vi "GE 5565PIORC.Registers.DMASIZ0.DMA Transfer Size.Set.vi"(8 "error in (no error)":errorcluster, 10 "DMA Transfer Size (Bytes)":u32, 11 "GE 5565PIORC in":refnum<class "GE 5565PIORC.lvclass">) -> (0 "error out":errorcluster, 3 "GE 5565PIORC out":refnum<class "GE 5565PIORC.lvclass">)   [LabVIEW 2017, in "GE 5565PIORC.lvclass"]
doc: "Indicates the number of bytes to transfer during a DMA operation."
uses:
  GE 5565PIORC.lvclass
  GE 5565PIORC.Registers.Local Configuration.ctl
  GE 5565PIORC.lvclass/GE 5565PIORC.ctl
  GE 5565PIORC.Registers.Local Configuration.Read (U32).vi
  GE 5565PIORC.Registers.Local Configuration.Write (U32).vi
  Methods/GE 5565PIORC.Registers.Read.vi
  Methods/GE 5565PIORC.Registers.Read (U32).vi
  Methods/GE 5565PIORC.Registers.Write.vi
  Methods/GE 5565PIORC.Registers.Write (U32).vi
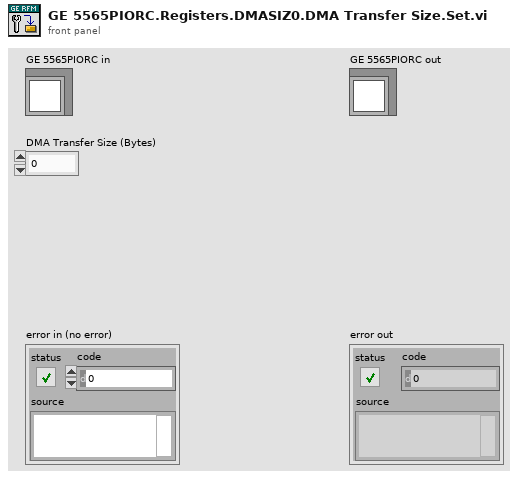
[diagram p1: front panel]
types:
  T1 = typedef "GE 5565PIORC.lvclass/GE 5565PIORC.Registers.Local Configuration.ctl" = u32
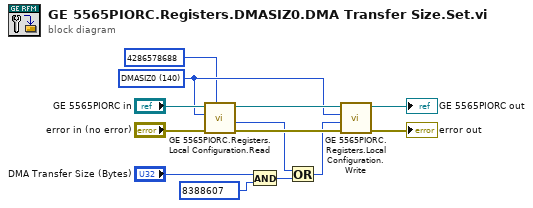
[diagram p0: block diagram]
diagram:
  w7 = T1 140 items=["MARBR"=8, "BIGEND"=12, "INTCSR"=104, "PCIHREV"=116, "DMAMODE0"=128, "DMAPADR0"=132, "DMALADR0"=136, "DMASIZ0"=140, "DMADPR0"=144, "DMACSR0"=168, "DMADAC0"=180, "LAS1RR"=240, "LAS1BA"=244] ("Local Configuration Registers")
  n1 = call-poly "GE 5565PIORC.Registers.Local Configuration.Read.vi"("Mask (0xFFFFFFFF)"=u32 4286578688, "error in (no error)"="error in (no error)", "Register"=w7, "GE 5565PIORC in"="GE 5565PIORC in") -> ("error out"=w13:errorcluster, "Value"=w3:u32, "GE 5565PIORC out"=w10:refnum<class "GE 5565PIORC.lvclass">)  [unwired: 5 in]
  n2 = And(x="DMA Transfer Size (Bytes)", y=u32 8388607 ("Mask (0xFFFFFFFF)")) -> (x .and. y?=w1:u32)
  n3 = Or(x=w3, y=w1) -> (x .or. y?=w2:u32)
  n4 = call-poly "GE 5565PIORC.Registers.Local Configuration.Write.vi"("error in (no error)"=w13, "Value"=w2, "Register"=w7, "GE 5565PIORC in"=w10) -> ("error out"=→"error out":errorcluster, "GE 5565PIORC out"=→"GE 5565PIORC out":refnum<class "GE 5565PIORC.lvclass">)  [unwired: 6 in]
